vi "matlab_TI2_shutdown.vi"(8 "error in":errorcluster) -> (0 "error out":errorcluster)   [LabVIEW 2018]
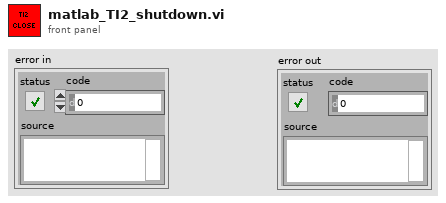
[diagram p1: front panel]
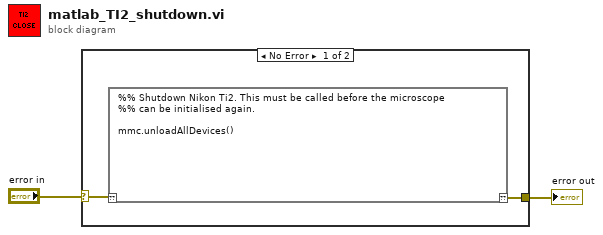
[diagram p0: block diagram]
diagram:
  n1 = case shown="No Error" "error in" {
    selector: "error in" -> [w4 w5]
    tunnel: [w3 w5] -> w1
    frame No Error {
      n2 = script code="%% Shutdown Nikon Ti2. This must be called before the microscope \n%% can be initialised again.\n\nmmc.unloadAllDevices()"("??"=w4) -> ("??"=w3:errorcluster)
    }
    frame Error {
    }
  }
  "error out" <- w1
